vi "Main.vi"(11 "Module Admin":refnum<class "Delacor_lib_QMH_Module Admin.lvclass">) -> ()   [LabVIEW 2019, in "PF_trial_1.lvlib"]
doc: "This template is based off of the Queued Message Handler design pattern and the Queued Message Handler project template that ships with LabVIEW.\n\nThe main difference is that the queue is private to this module and communication between modules is performed via Broadcast and Request events.\n\nRequest events are wrapped in public API methods and are handled in the Event Handling Loop (EHL) of this VI. Any module can register for Broadcast events sent by this module. The EHL generates messages based on user interface actions.\n\nThe Message Handling Loop (MHL) processes messages generated by the EHL, or by other messages. The messages are string values, so new messages can be added easily to the Message Cases case structure in the MHL. Each message cluster can also provide an optional value for Message Data, which is a variant that can be converted to whatever message-specific data is required.\n_____\nBased on Delacor QMH Project Template 5.0.0.82."
uses:
  PF_trial_1.lvlib
  <vilib>/Delacor/Delacor QMH/Libraries/Module Admin_class/Delacor_lib_QMH_Module Admin.lvclass
  Module Data--cluster.ctl
  <vilib>/Delacor/Delacor QMH/Libraries/Message Queue_class/Delacor_lib_QMH_Message Queue.lvclass/Delacor_lib_QMH_Message Queue.ctl
  Stop Argument--cluster.ctl
  <vilib>/Delacor/Delacor QMH/Libraries/Module Admin_class/Delacor_lib_QMH_Module Admin.lvclass/Delacor_lib_QMH_Module Admin.ctl
  <vilib>/Utility/miscctls.llb/LVPointTypeDef.ctl
  <vilib>/Delacor/Delacor QMH/Libraries/Message Queue_class/Delacor_lib_QMH_Enqueue Message (Single).vi
  <vilib>/Delacor/Delacor QMH/Libraries/Module Admin_class/Delacor_lib_QMH_Get External Launch.vi
  <vilib>/Utility/error.llb/Error Cluster From Error Code.vi
  Global 1.vi
  <vilib>/ErrorRing/Error Ring.xnode
  <vilib>/Delacor/Delacor QMH/Libraries/Message Queue_class/Delacor_lib_QMH_Message Queue.lvclass
panel:
  out "Waveform Chart":dbl(graph)
  out "Gauge On?":bool
  in  "Get Status":bool
  in  "tpg361_delay":u32=50
  out "Error Status":string
  in  "Error status":bool
  out "Reset Status":string
  in  "Reset":bool
  in  "Gauge On-Off":enum16{"NO CHANGE", "OFF", "ON"}(ring)
  out "UNIT":string
  in  "Serial Settings:End Mode for Reads":u16(ring) items=["None", "Last Bit", "TermChar"]
  in  "Serial Settings:End Mode for Writes":u16(ring) items=["None", "Last Bit", "TermChar", "Break"]
  in  "Serial Settings:Baud Rate":u32(ring)=9600 items=["9.6KHz"=9600, "19.2KHz"=19200]
  in  "tpg_visa":refnum<visa-resource-name>
  out "Gauge Type":string
  in  "Get Gauge":bool
  in  "SETTING UNIT":T1(ring)=enum."Torr"
  in  "Acquisition time":i32=2000
  out "Pressure (Torr)":string
  in  "Get Pressure":bool
  in  "Simulate MHL Error":bool
  in  "Simulate EHL Error":bool
  out "error out":errorcluster
  out "Status":string
  # "RESET STATUS:\n0 = No Error\n1 = Watchdog has responded\n2 = Task Fail Error\n5 = FLASH Error\n6 = RAM Error\n7 = EEPROM Error\n9 = DISPLAY Error\n10 = A/D Converter Error\n11 = Gauge Error\n12 = Gauge Identification Error"
  # "ERROR STATUS:\n0000 = No Error\n1000 = ERROR (controller error (see display on front\npanel)\n0100 = NO HWR (no hardware) \n0010 = PAR (inadmissible parameter) \n0001 = SYN (Syntax error)"
  # "INITIALIZATION:"
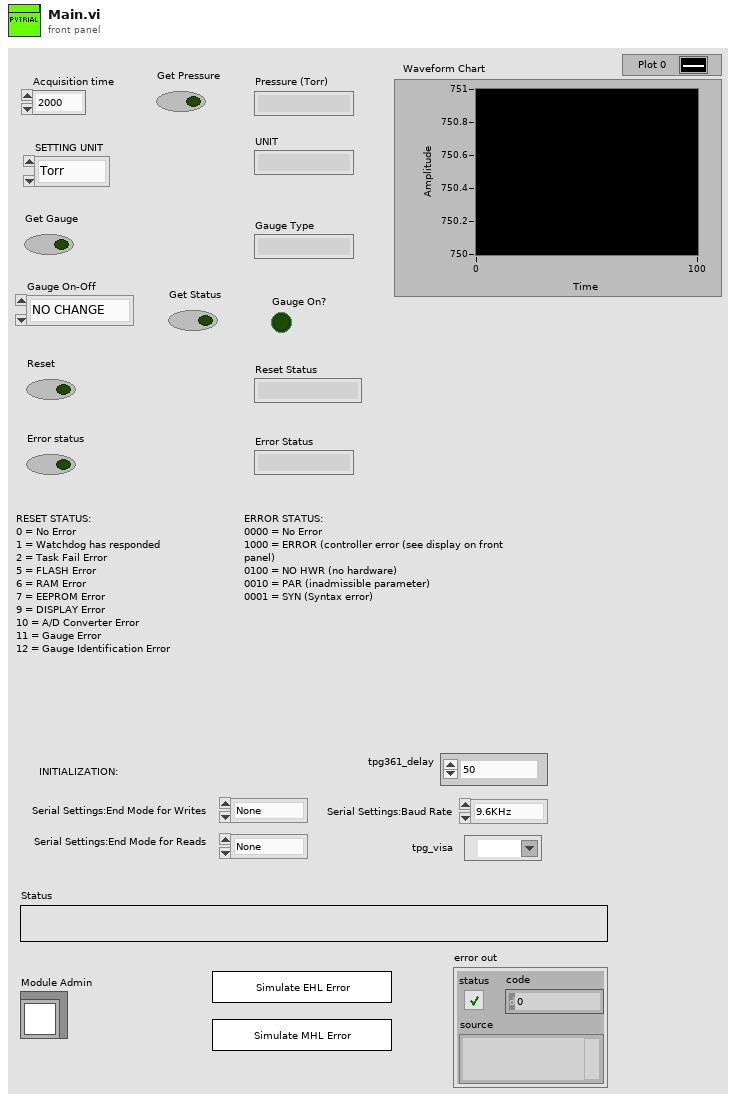
[diagram p1: front panel]
types:
  T1 = enum16{"mBar", "Torr", "Pascal", "micron", "hPascal", "Volt"}
  T2 = typedef "PF_trial_1.lvlib/Request Events--cluster.ctl" = cluster{"Stop Module":refnum<user-event>, "Show Panel":refnum<user-event>, "Hide Panel":refnum<user-event>, "Get Module Execution Status":refnum<user-event>, "Show Diagram":refnum<user-event>}
  T3 = typedef "PF_trial_1.lvlib/Module Data--cluster.ctl" = cluster{"Status":string}
  T4 = enum32{"invalid lock state", "Not Locked", "Locked (No Password)", "Password-protected"}
  T5 = typedef "PF_trial_1.lvlib/Stop Argument--cluster.ctl" = cluster{"Origin":string, "Exit via Stop Module Req?":bool, "Wait for Module to stop?":bool}
  T6 = typedef "LVPointTypeDef.ctl" = cluster{"Horizontal":i16, "Vertical":i16}
  T7 = enum32{"Invalid", "Standard", "Closed", "Hidden", "Minimized", "Maximized"}
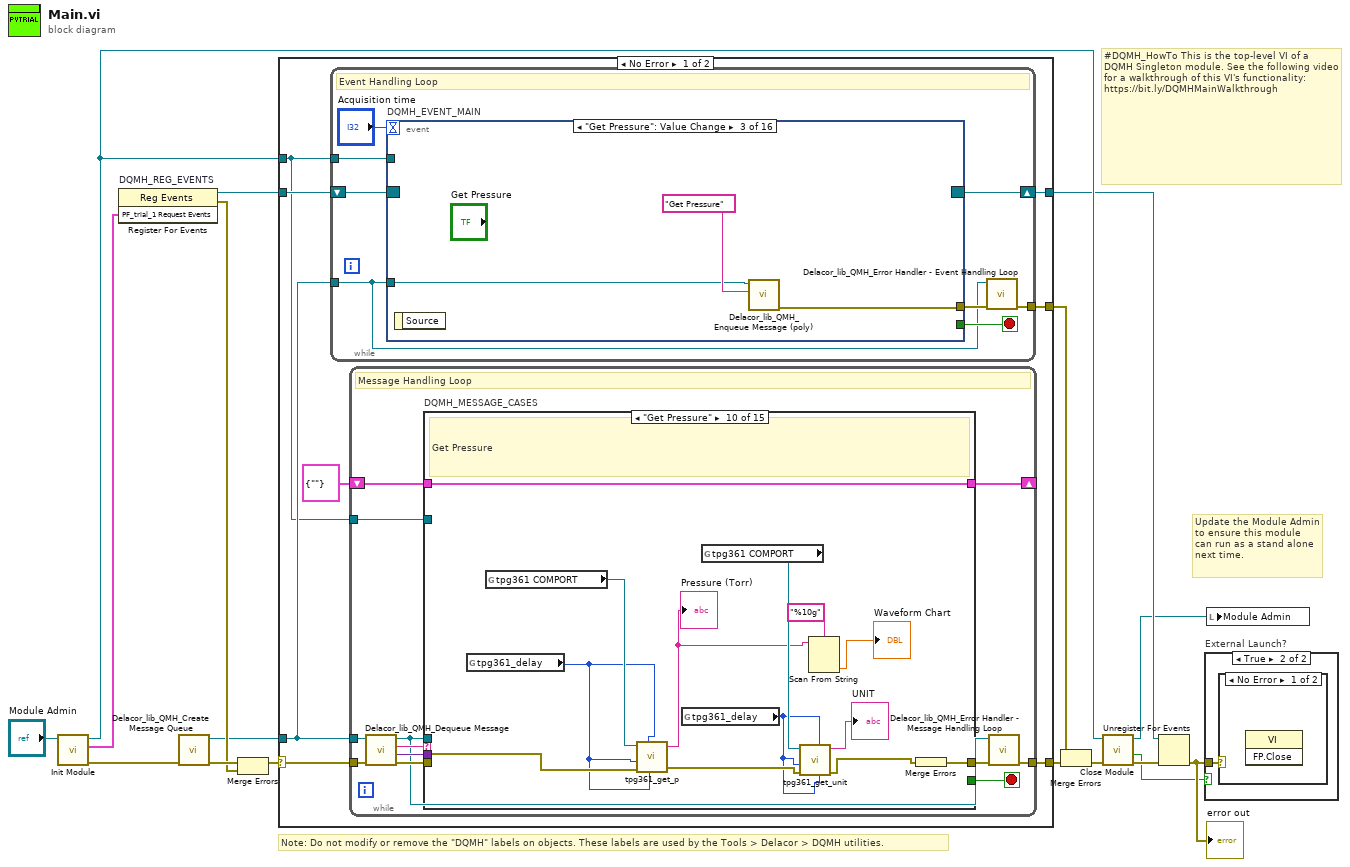
[diagram p0: block diagram]
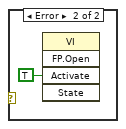
[diagram p3: hidden frame]
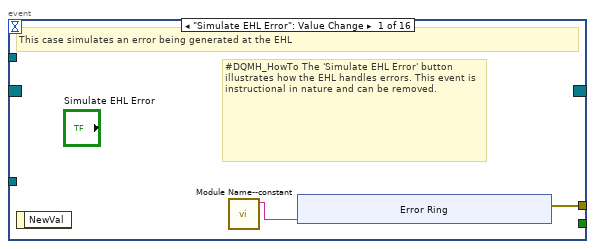
[diagram p4: hidden frame]
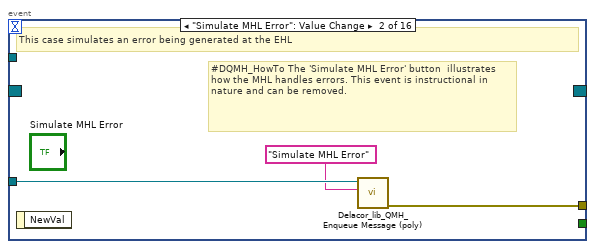
[diagram p5: hidden frame]
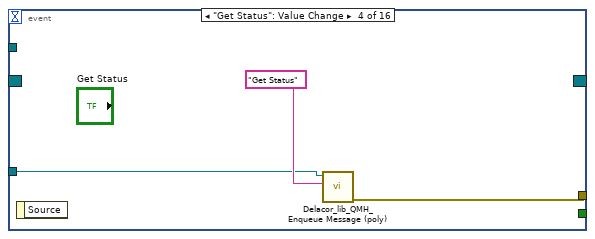
[diagram p6: hidden frame]
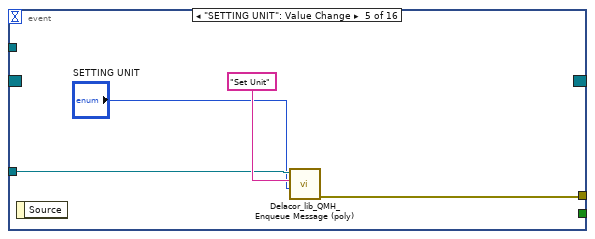
[diagram p7: hidden frame]
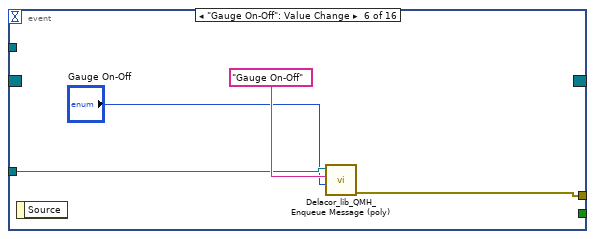
[diagram p8: hidden frame]
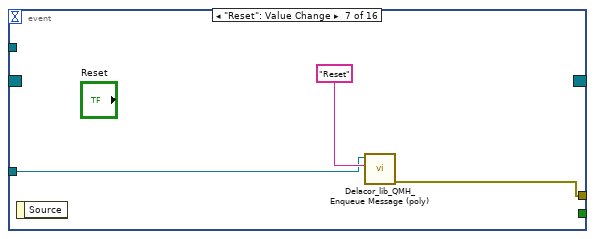
[diagram p9: hidden frame]
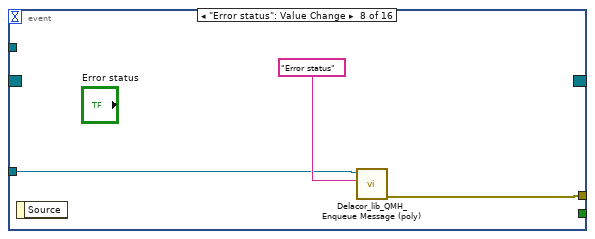
[diagram p10: hidden frame]
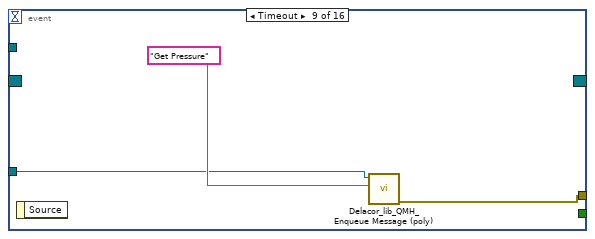
[diagram p11: hidden frame]
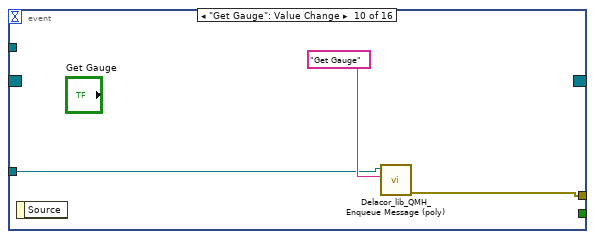
[diagram p12: hidden frame]
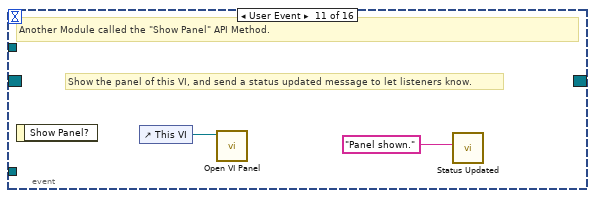
[diagram p13: hidden frame]
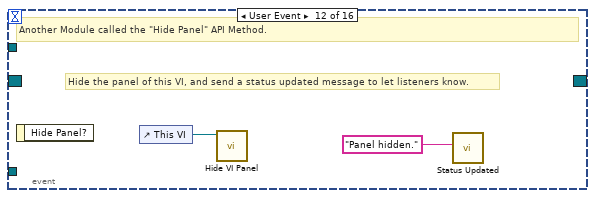
[diagram p14: hidden frame]
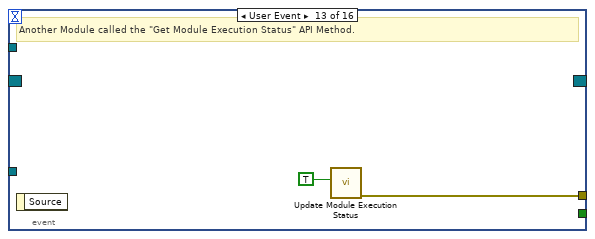
[diagram p15: hidden frame]
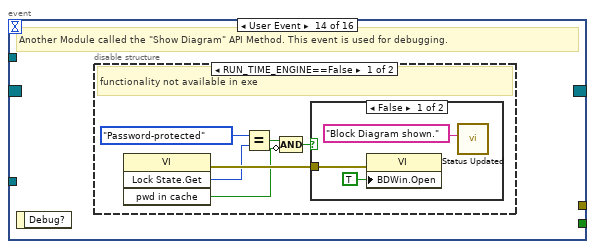
[diagram p16: hidden frame]
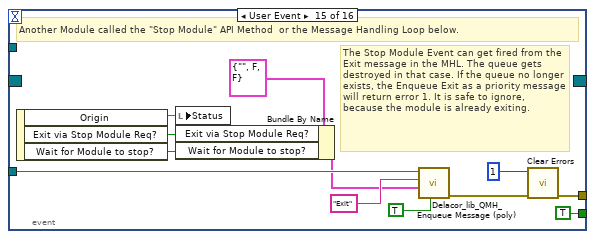
[diagram p19: hidden frame]
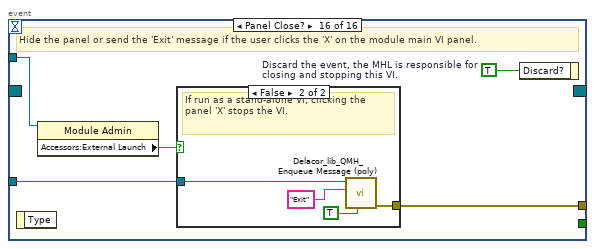
[diagram p20: hidden frame]
diagram:
  # "#DQMH_HowTo This is the top-level VI of a DQMH Singleton module. See the following video for a walkthrough of this VI's functionality: https://bit.ly/DQMHMainWalkthrough"
  # "Note: Do not modify or remove the \"DQMH\" labels on objects. These labels are used by the Tools > Delacor > DQMH utilities."
  # "Update the Module Admin to ensure this module can run as a stand alone next time."
  n1 = call "Init Module.vi"("Singleton Module Admin in"="Module Admin") -> ("error out"=w16:errorcluster, "PF_trial_1 Request Events"=w5:T2, "Singleton Module Admin out"=w8:refnum<class "Delacor_lib_QMH_Module Admin.lvclass">)  [unwired: 8 in]
  n2 = register-events "DQMH_REG_EVENTS"(w5) -> (reference out=w6:refnum<event-registration>, error out=w9:errorcluster)  [unwired: 2 in]
  n3 = call <vilib>:"Delacor_lib_QMH_Create Message Queue.vi"("error in (no error)"=w16) -> ("error out"=w11:errorcluster, "Message Queue"=w4:refnum<class "Delacor_lib_QMH_Message Queue.lvclass">)  [unwired: 9 in]
  n4 = Merge Errors(w11, w9) -> (w10:errorcluster)
  n5 = case shown="No Error" w10 {
    selector: w10 -> [w23 w273]
    tunnel: [w25 w272] -> w17
    tunnel: [w22 w278] -> w7
    tunnel: w6 -> [w20 w278]
    tunnel: w4 -> [w19 w271]
    tunnel: [w24 _] -> w14
    tunnel: w8 -> [w18 w274]
    frame No Error {
      n6 = while {
        tunnel: w19 -> [w27]
        shift-right: [w30] -> w22
        shift-left: w20 -> [w31]
        tunnel: [w32] -> w24
        tunnel: w18 -> [w28]
        stop <- w29 stop-if-true
        # "Event Handling Loop"
        n7 = event "DQMH_EVENT_MAIN" shown="[2] \"Get Pressure\": Value Change" {
          selector: w31 -> [_ _ _ _ _ _ _ _ _ _ _ _ _ _ _ _]
          dyn-events: [_ _ _ _ _ _ _ _ _ _ _ _ _ _ _ _] -> w30
          timeout: "Acquisition time" -> [_ _ _ _ _ _ _ _ _ _ _ _ _ _ _ _]
          tunnel: [_ _ _ _ _ _ _ _ _ _ _ _ _ _ TRUE ("Discard?") _] -> w29
          tunnel: w27 -> [_ w44 w47 w50 w54 w58 w60 w64 w67 w70 _ _ _ _ w94 w101]
          tunnel: [w35 w45 w46 w49 w53 w56 w61 w63 w66 w69 _ _ w77 _ w97 w103] -> w33
          tunnel: w28 -> [_ _ _ _ _ _ _ _ _ _ _ _ _ _ _ w100]
          event "Simulate EHL Error": Value Change {
            # "#DQMH_HowTo The 'Simulate EHL Error' button  illustrates how the EHL handles errors. This event is instructional in nature and can be removed."
            # "This case simulates an error being generated at the EHL"
            n8 = event-data() -> ()  [unwired: 1 in, 1 out]
            n9 = call "Module Name--constant.vi"() -> ("Module Name"=w34:string)  [unwired: 11 in]
            n10 = xnode "Error Ring"("parameter 0"=w34) -> ("error out"=w35:errorcluster)
          }
          event "Simulate MHL Error": Value Change {
            # "#DQMH_HowTo The 'Simulate MHL Error' button  illustrates how the MHL handles errors. This event is instructional in nature and can be removed."
            # "This case simulates an error being generated at the EHL"
            n11 = event-data() -> ()  [unwired: 1 in, 1 out]
            n12 = call-poly <vilib>:"Delacor_lib_QMH_Enqueue Message (poly).vi"("Message"="Simulate MHL Error", "Message Queue in"=w44) -> ("error out"=w45:errorcluster)  [unwired: 8 in, 1 out]
          }
          event "Get Pressure": Value Change {
            n13 = event-data() -> ()  [unwired: 1 in, 1 out]
            n14 = call-poly <vilib>:"Delacor_lib_QMH_Enqueue Message (poly).vi"("Message"="Get Pressure", "Message Queue in"=w47) -> ("error out"=w46:errorcluster)  [unwired: 8 in, 1 out]
          }
          event "Get Status": Value Change {
            n15 = event-data() -> ()  [unwired: 1 in, 1 out]
            n16 = call-poly <vilib>:"Delacor_lib_QMH_Enqueue Message (poly).vi"("Message"="Get Status", "Message Queue in"=w50) -> ("error out"=w49:errorcluster)  [unwired: 8 in, 1 out]
          }
          event "SETTING UNIT": Value Change {
            n17 = event-data() -> ()  [unwired: 1 in, 1 out]
            n18 = call-poly <vilib>:"Delacor_lib_QMH_Enqueue Message (poly).vi"("Message Data"="SETTING UNIT", "Message"="Set Unit", "Message Queue in"=w54) -> ("error out"=w53:errorcluster)  [unwired: 7 in, 1 out]
          }
          event "Gauge On-Off": Value Change {
            n19 = event-data() -> ()  [unwired: 1 in, 1 out]
            n20 = call-poly <vilib>:"Delacor_lib_QMH_Enqueue Message (poly).vi"("Message Data"="Gauge On-Off", "Message"="Gauge On-Off", "Message Queue in"=w58) -> ("error out"=w56:errorcluster)  [unwired: 7 in, 1 out]
          }
          event "Reset": Value Change {
            n21 = event-data() -> ()  [unwired: 1 in, 1 out]
            n22 = call-poly <vilib>:"Delacor_lib_QMH_Enqueue Message (poly).vi"("Message"="Reset", "Message Queue in"=w60) -> ("error out"=w61:errorcluster)  [unwired: 8 in, 1 out]
          }
          event "Error status": Value Change {
            n23 = event-data() -> ()  [unwired: 1 in, 1 out]
            n24 = call-poly <vilib>:"Delacor_lib_QMH_Enqueue Message (poly).vi"("Message"="Error status", "Message Queue in"=w64) -> ("error out"=w63:errorcluster)  [unwired: 8 in, 1 out]
          }
          event Timeout {
            n25 = event-data() -> ()  [unwired: 1 in, 1 out]
            n26 = call-poly <vilib>:"Delacor_lib_QMH_Enqueue Message (poly).vi"("Message"="Get Pressure", "Message Queue in"=w67) -> ("error out"=w66:errorcluster)  [unwired: 8 in, 1 out]
          }
          event "Get Gauge": Value Change {
            n27 = event-data() -> ()  [unwired: 1 in, 1 out]
            n28 = call-poly <vilib>:"Delacor_lib_QMH_Enqueue Message (poly).vi"("Message"="Get Gauge", "Message Queue in"=w70) -> ("error out"=w69:errorcluster)  [unwired: 8 in, 1 out]
          }
          event User Event {
            # "Show the panel of this VI, and send a status updated message to let listeners know."
            # "Another Module called the \"Show Panel\" API Method."
            n29 = event-data() -> ()  [unwired: 1 in, 1 out]
            n30 = control-ref of="This VI"() -> (w73:refnum<vi>)
            n31 = call "Open VI Panel.vi"("VI"=w73) -> ()  [unwired: 10 in, 1 out]
            n32 = call "Status Updated.vi"("Status"="Panel shown." ("format string")) -> ()  [unwired: 10 in, 1 out]
          }
          event User Event {
            # "Hide the panel of this VI, and send a status updated message to let listeners know."
            # "Another Module called the \"Hide Panel\" API Method."
            n33 = event-data() -> ()  [unwired: 1 in, 1 out]
            n34 = control-ref of="This VI"() -> (w75:refnum<vi>)
            n35 = call "Hide VI Panel.vi"("VI"=w75) -> ()  [unwired: 10 in, 1 out]
            n36 = call "Status Updated.vi"("Status"="Panel hidden." ("format string")) -> ()  [unwired: 10 in, 1 out]
          }
          event User Event {
            # "Another Module called the \"Get Module Execution Status\" API Method."
            n37 = event-data() -> ()  [unwired: 1 in, 1 out]
            n38 = call "Update Module Execution Status.vi"("Running?"=TRUE) -> ("error out"=w77:errorcluster)  [unwired: 10 in]
          }
          event User Event {
            # "Another Module called the \"Show Diagram\" API Method. This event is used for debugging."
            n39 = event-data() -> ()  [unwired: 1 in, 1 out]
            n40 = disable-structure shown="RUN_TIME_ENGINE==False" {
              frame condition #0 (active) {
                # "functionality not available in exe"
                n41 = invoke class="VI" method="Lock State.Get"() -> (error out=w83:errorcluster, "Get Lock State"=w82:T4, "pwd in cache"=w79:bool)  [unwired: 4 in, 1 out]
                n42 = Equal?(x=T4."Password-protected", y=w82) -> (x = y?=w80:bool)
                n43 = Compound Arithmetic op=AND(w80, invert w79) -> (w78:bool)
                n44 = case shown="False" w78 {
                  tunnel: w83 -> [w86 _]
                  frame False {
                    n45 = property class="VI"(error in=w86, "BDWin.Open"=TRUE ("Block Diagram Window:Open")) -> ()  [unwired: 1 in, 2 out]
                    n46 = call "Status Updated.vi"("Status"="Block Diagram shown." ("format string")) -> ()  [unwired: 10 in, 1 out]
                  }
                  frame True {
                    # "Password-protected VI, and the password is not in the cache. Do not show the diagram."
                  }
                }
              }
              frame condition #1 {
              }
            }
          }
          event User Event {
            # "The Stop Module Event can get fired from the Exit message in the MHL. The queue gets destroyed in that case. If the queue no longer exists, the Enqueue Exit as a priority message will return error 1. It is safe to ignore, because the module is already exiting."
            # "Another Module called the \"Stop Module\" API Method  or the Message Handling Loop below."
            n47 = event-data() -> ("Origin"=w93:string, "Exit via Stop Module Req?"=w89:bool, "Wait for Module to stop?"=w88:bool)  [unwired: 1 in]
            n48 = local write "Status"(w93) -> ()
            n49 = Bundle By Name(cluster=T5 {"Origin"="", "Exit via Stop Module Req?"=FALSE, "Wait for Module to stop?"=FALSE} ("Stop Argument"), "Exit via Stop Module Req?"=w89, "Wait for Module to stop?"=w88) -> (w87:T5)
            n50 = call-poly <vilib>:"Delacor_lib_QMH_Enqueue Message (poly).vi"("Priority Message? (F)"=TRUE, "Message Data"=w87, "Message"="Exit", "Message Queue in"=w94) -> ("error out"=w98:errorcluster)  [unwired: 6 in, 1 out]
            n51 = call <vilib>:"Clear Errors.vi"("error in (no error)"=w98, "specific error code to clear (0: all)"=1) -> ("error out"=w97:errorcluster)  [unwired: 4 in, 1 out]
          }
          event Panel Close? {
            w102 = TRUE  # Discard the event, the MHL is responsible for closing and stopping this VI.
            # "Hide the panel or send the 'Exit' message if the user clicks the 'X' on the module main VI panel."
            n52 = event-data() -> ()  [unwired: 1 in, 1 out]
            n53 = property class="Module Admin"(reference=w100) -> ("Accessors:External Launch"=w99:bool)  [unwired: 1 in, 2 out]
            n54 = case shown="False" w99 {
              tunnel: w101 -> [_ w107]
              tunnel: [_ w108] -> w103
              frame True {
                # "If externally launched, clicking the 'X' hides the panel, but doesn't close it."
                n55 = control-ref of="This VI"() -> (w104:refnum<vi>)
                n56 = call "Hide VI Panel.vi"("VI"=w104) -> ()  [unwired: 10 in, 1 out]
              }
              frame False {
                # "If run as a stand-alone VI, clicking the panel 'X' stops the VI."
                n57 = call-poly <vilib>:"Delacor_lib_QMH_Enqueue Message (poly).vi"("Priority Message? (F)"=TRUE, "Message"="Exit", "Message Queue in"=w107) -> ("error out"=w108:errorcluster)  [unwired: 7 in, 1 out]
              }
            }
            n58 = event-data("Discard?"=w102) -> ()  [unwired: 1 in, 1 out]
          }
        }
        n59 = call-dynamic "Delacor_lib_QMH_Error Handler - Event Handling Loop.vi"("error in (no error)"=w33, "Message Queue in"=w27) -> ("dup error in"=w32:errorcluster)  [unwired: 8 in, 1 out]
      }
      n60 = while {
        tunnel: w19 -> [w111]
        shift-right: [w115] -> _
        shift-left: T3 {"Status"=""} ("Data Cluster") -> [w116]
        tunnel: w23 -> [w119]
        tunnel: [w117] -> w25
        tunnel: w18 -> [w109]
        stop <- w114 stop-if-true
        # "Message Handling Loop"
        n61 = call-dynamic "Delacor_lib_QMH_Dequeue Message.vi"("error in (no error)"=w119, "Message Queue in"=w111) -> ("error out"=w118:errorcluster, "Message Data"=w112:variant, "Message"=w113:string, "Message Queue out"=w110:refnum<class "Delacor_lib_QMH_Message Queue.lvclass">)  [unwired: 6 in]
        n62 = case "DQMH_MESSAGE_CASES" shown="\"Get Pressure\"" w113 {
          selector: w113 -> [_ _ _ _ _ _ _ _ _ _ _ _ _ _ w258]
          tunnel: w110 -> [_ _ _ _ _ _ _ _ _ _ _ _ w226 w251 _]
          tunnel: w118 -> [w144 w148 w151 w154 w162 w168 w177 w183 w192 w206 w210 w215 w233 w256 w260]
          tunnel: [w143 w148 w150 w158 w164 w170 w179 w185 w195 w208 w210 w214 w229 w254 w261] -> w120
          tunnel: w116 -> [w134 w147 w149 w157 w163 w169 w178 w184 w194 w207 w209 w212 w228 w250 w259]
          tunnel: [w133 w147 w149 w157 w163 w169 w178 w184 w194 w207 w209 w212 w228 w250 w259] -> w115
          tunnel: [_ _ _ _ _ _ _ _ _ _ _ _ _ w249 _] -> w114
          tunnel: w112 -> [_ _ _ _ _ _ w174 _ w190 _ _ _ w227 w248 _]
          tunnel: w109 -> [w135 _ _ _ _ _ _ _ _ _ _ _ w225 w243 _]
          frame "Initialize" {
            w128 = "Initial Message" ("Initial Message")
            # "#CodeNeeded - Initialize the appearance of the front panel."
            # "Initialize - Any operation that needs to be done before the module can receive messages. Synchronize Caller Events.vi will inform Start Module.vi that the module has launched and is ready to receive messages. Module Did Init.vi will broadcast that the module initialized."
            n63 = call "Synchronize Caller Events.vi"("error in (no error)"=w144, "Singleton Module Admin in"=w135) -> ("error out"=w127:errorcluster, "Singleton Module Admin out"=w130:refnum<class "Delacor_lib_QMH_Module Admin.lvclass">)  [unwired: 8 in]
            n64 = property class="Module Admin"(reference=w130) -> ("Accessors:External Launch"=w139:bool)  [unwired: 1 in, 2 out]
            n65 = global write "Global 1.vi" "tpg361_delay"("tpg361_delay") -> ()
            n66 = global write "Global 1.vi" "tpg361 COMPORT"("tpg_visa") -> ()
            n67 = Select(t=T7."Hidden" ("State"), s=w139, f=T7."Standard" ("State")) -> (s? t:f=w136:T7)
            n68 = call "tpg361_visa_init.vi"("thcd_visa"="tpg_visa", "err_in"=w127, "Serial Settings:Baud Rate"="Serial Settings:Baud Rate", "Serial Settings:End Mode for Writes"="Serial Settings:End Mode for Writes", "Serial Settings:End Mode for Reads"="Serial Settings:End Mode for Reads") -> ("err_out"=w126:errorcluster)  [unwired: 1 out]
            n69 = call "Module Name--constant.vi"() -> ("Module Name"=w142:string)  [unwired: 11 in]
            n70 = property class="VI"("Front Panel.Title"=w142) -> (reference out=w141:refnum<vi>, error out=w146:errorcluster)  [unwired: 2 in]
            n71 = call "Module Name--constant.vi"() -> ("Module Name"=w131:string)  [unwired: 11 in]
            n72 = invoke class="VI" method="FP.Open"(reference=w141, error in=w146, "State"=w136) -> (reference out=w140:refnum<vi>, error out=w145:errorcluster)  [unwired: 2 in, 3 out]
            n73 = Bundle By Name(cluster=w134, "Status"=w128) -> (w133:T3)
            n74 = call "Module Did Init.vi"("error in (no error)"=w126, "Initialized?"=TRUE, "Origin"=w131) -> ("error out"=w143:errorcluster)  [unwired: 8 in]
            n75 = invoke class="VI" method="FP.Center"(reference=w140, error in=w145) -> ()  [unwired: 1 in, 3 out]
            n76 = property on="Pane" class="Pane"("Origin"=T6 {"Horizontal"=0, "Vertical"=0}) -> ()  [unwired: 2 in, 2 out]
            "Status" <- w128
          }
          frame "--- Module Specific ---" {
            # "Separator -- The following cases handle messages specific to this Module."
          }
          frame "---Copy This Frame---" {
            # "Duplicate this frame when creating new messages.  Change this comment in the duplicated frame to describe this message."
            n77 = Merge Errors(w151) -> (w150:errorcluster)
          }
          frame "Get Status" {
            # "Duplicate this frame when creating new messages.  Change this comment in the duplicated frame to describe this message."
            n78 = global read "Global 1.vi" "tpg361 COMPORT"() -> (w155:refnum<visa-resource-name>)
            n79 = global read "Global 1.vi" "tpg361_delay"() -> (w152:u32)
            n80 = call "tpg361_get_status.vi"("tpg361_delay 3"=w152, "tpg361_delay 2"=w152, "err_in"=w154, "tpg361_delay"=w152, "tpg361_visa"=w155) -> ("err_out"=w153:errorcluster, "Gauge status"=→"Gauge On?":bool)  [unwired: 4 in]
            n81 = Merge Errors(w153) -> (w158:errorcluster)
          }
          frame "Error status" {
            # "Duplicate this frame when creating new messages.  Change this comment in the duplicated frame to describe this message."
            n82 = global read "Global 1.vi" "tpg361 COMPORT"() -> (w160:refnum<visa-resource-name>)
            n83 = call "tpg361_ERR.vi"("err_in"=w162, "tpg361_visa"=w160) -> ("err_out"=w161:errorcluster, "Error Status"=→"Error Status":string)  [unwired: 7 in]
            n84 = Merge Errors(w161) -> (w164:errorcluster)
          }
          frame "Reset" {
            # "Duplicate this frame when creating new messages.  Change this comment in the duplicated frame to describe this message."
            n85 = global read "Global 1.vi" "tpg361 COMPORT"() -> (w166:refnum<visa-resource-name>)
            n86 = call "tpg361_reset.vi"("err_in"=w168, "tpg361_visa"=w166) -> ("err_out"=w167:errorcluster, "Error Status"=→"Reset Status":string)  [unwired: 7 in]
            n87 = Merge Errors(w167) -> (w170:errorcluster)
          }
          frame "Gauge On-Off" {
            # "Duplicate this frame when creating new messages.  Change this comment in the duplicated frame to describe this message."
            n88 = Variant To Data(error in=w177, Variant=w174) -> (data=w173:enum16{"NO CHANGE", "OFF", "ON"}, error out=w176:errorcluster)  [unwired: 1 in]
            n89 = global read "Global 1.vi" "tpg361_delay"() -> (w172:u32)
            n90 = global read "Global 1.vi" "tpg361 COMPORT"() -> (w175:refnum<visa-resource-name>)
            n91 = call "tpg361_on_off.vi"("tpg361_delay 3"=w172, "tpg361_delay 2"=w172, "err_in"=w176, "tpg361_delay"=w172, "Gauge On-Off"=w173, "tpg361_visa"=w175) -> ("err_out"=w171:errorcluster)  [unwired: 3 in, 1 out]
            n92 = Merge Errors(w171) -> (w179:errorcluster)
          }
          frame "Get Gauge" {
            # "Duplicate this frame when creating new messages.  Change this comment in the duplicated frame to describe this message."
            n93 = global read "Global 1.vi" "tpg361 COMPORT"() -> (w180:refnum<visa-resource-name>)
            n94 = call "tpg361_get_gauge.vi"("err_in"=w183, "tpg361_visa"=w180) -> ("err_out"=w182:errorcluster, "Gauge Type"=→"Gauge Type":string)  [unwired: 7 in]
            n95 = Merge Errors(w182) -> (w185:errorcluster)
          }
          frame "Set Unit" {
            # "Set Unit"
            n96 = global read "Global 1.vi" "tpg361_delay"() -> (w186:u32)
            n97 = Variant To Data(error in=w192, type=T1."Torr", Variant=w190) -> (data=w189:T1, error out=w191:errorcluster)
            n98 = global read "Global 1.vi" "tpg361 COMPORT"() -> (w187:refnum<visa-resource-name>)
            n99 = call "tpg361_set_unit.vi"("tpg361_delay 3"=w186, "tpg361_delay 2"=w186, "err_in"=w191, "tpg361_delay"=w186, "tpg361_visa"=w187, "SETTING UNIT"=w189) -> ("err_out"=w193:errorcluster)  [unwired: 4 in]
            n100 = Merge Errors(w193) -> (w195:errorcluster)
          }
          frame "Get Pressure" {
            # "Get Pressure"
            n101 = global read "Global 1.vi" "tpg361_delay"() -> (w204:u32)
            n102 = global read "Global 1.vi" "tpg361 COMPORT"() -> (w205:refnum<visa-resource-name>)
            n103 = call "tpg361_get_p.vi"("tpg361_delay 3"=w204, "err_in"=w206, "tpg361_delay"=w204, "tpg361_delay 2"=w204, "tpg361_visa"=w205) -> ("err_out"=w203:errorcluster, "Pressure (Torr)"=w198:string)  [unwired: 4 in]
            "Pressure (Torr)" <- w198
            n104 = global read "Global 1.vi" "tpg361_delay"() -> (w200:u32)
            n105 = global read "Global 1.vi" "tpg361 COMPORT"() -> (w201:refnum<visa-resource-name>)
            n106 = call "tpg361_get_unit.vi"("tpg361_visa"=w201, "tpg361_delay"=w200, "err_in"=w203, "tpg361_delay 2"=w200, "tpg361_delay 3"=w200) -> ("UNIT"=→"UNIT":string, "err_out"=w202:errorcluster)  [unwired: 3 in]
            n107 = Scan From String(format string="%10g", input string=w198) -> (output 1=→"Waveform Chart":dbl)  [unwired: 3 in, 3 out]
            n108 = Merge Errors(w202) -> (w208:errorcluster)
          }
          frame "--- Exit and Error Handling---" {
            # "Separator - The following cases handle errors and exit messages."
          }
          frame "Simulate MHL Error" {
            # "#DQMH_HowTo The 'Simulate MHL Error' button  illustrates how the MHL handles errors. This event is instructional in nature and can be removed."
            # "Simulate an error occurring at the MHL"
            n109 = call "Module Name--constant.vi"() -> ("Module Name"=w211:string)  [unwired: 11 in]
            n110 = xnode "Error Ring"("parameter 0"=w211) -> ("error out"=w213:errorcluster)
            n111 = Merge Errors(w215, w213) -> (w214:errorcluster)
          }
          frame "Error" {
            # "#CodeRecommended - If you ever change the name of this \"Error\" message, you'll need to update the name in the Check Loop Error.vi as well."
            # "#CodeRecommended - If the module is running in standalone mode (External Launch = FALSE), this code will pop up an error dialog and call the 'Exit' message if an error occurs. Add more fine-grained error handling here."
            # "Error - Check the error message data and respond accordingly. This message is sent by the \"Error Handler\" VIs at the end of each loop in this application."
            n112 = property class="Module Admin"(reference=w225) -> ("Accessors:External Launch"=w224:bool)  [unwired: 1 in, 2 out]
            n113 = Variant To Data(error in=w233, type=errorcluster {"status"=FALSE, "code"=0, "source"=""} ("error constant"), Variant=w227) -> (data=w234:errorcluster, error out=w231:errorcluster)
            n114 = call "Module Name--constant.vi"() -> ("Module Name"=w223:string)  [unwired: 11 in]
            n115 = call "Error Reported.vi"("Additional Information"=w223, "Error"=w234) -> ()  [unwired: 9 in, 1 out]
            n116 = case shown="False" w224 {
              tunnel: [w239 _] -> w230
              tunnel: w226 -> [w237 _]
              tunnel: w234 -> [w238 _]
              frame False {
                # "If the module is running standalone, then pop up an error dialog and call the \"Exit\" message."
                n117 = call <vilib>:"Simple Error Handler.vi"("error in (no error)"=w238) -> ()  [unwired: 4 in, 5 out]
                n118 = call-poly <vilib>:"Delacor_lib_QMH_Enqueue Message (poly).vi"("Priority Message? (F)"=TRUE, "Message"="Exit", "Message Queue in"=w237) -> ("error out"=w239:errorcluster)  [unwired: 7 in, 1 out]
              }
              frame True {
                # "If the module was launched externally, calling the Error Reported broadcast VI is the only action performed by the \"Error\" message. The module's caller can then process the error appropriately."
              }
            }
            n119 = Merge Errors(w231, w230) -> (w229:errorcluster)
            n120 = local write "error out"(w229) -> ()
          }
          frame "Exit" {
            w247 = 91  # 91: not all Exit messages will have an argument
            w249 = TRUE  # Stop the VI
            # "Release the message queue reference"
            # "#CodeNeeded - Add any required cleanup code here"
            # "Exit - Exit the application."
            n121 = Variant To Data(error in=w256, type=T5 {"Origin"="", "Exit via Stop Module Req?"=FALSE, "Wait for Module to stop?"=FALSE} ("Stop Argument"), Variant=w248) -> (data=w245:T5, error out=w253:errorcluster)
            n122 = call <vilib>:"Clear Errors.vi"("error in (no error)"=w253, "specific error code to clear (0: all)"=w247) -> ("error out"=w255:errorcluster)  [unwired: 4 in, 1 out]
            n123 = global read "Global 1.vi" "tpg361 COMPORT"() -> (w240:refnum<visa-resource-name>)
            n124 = call-dynamic "Delacor_lib_QMH_Release Message Queue.vi"("error in (no error)"=w255, "Message Queue"=w251) -> ("error out"=w242:errorcluster)  [unwired: 9 in]
            n125 = control-ref of="This VI"() -> (w244:refnum<vi>)
            n126 = call "tpg361_visa_close.vi"("VISA session"=w240, "error in (no error)"=w242) -> ("error out"=w241:errorcluster)  [unwired: 13 in]
            n127 = call "Handle Exit.vi"("Stop Argument"=w245, "Admin in"=w243, "VI reference"=w244) -> ("error out"=w252:errorcluster)  [unwired: 7 in, 1 out]
            n128 = Merge Errors(w241, w252) -> (w254:errorcluster)
          }
          frame Default {
            # "'Default' case only runs if there is a message that isn't defined in any of the other cases.  Output a programming error."
            n129 = call "Module Name--constant.vi"() -> ("Module Name"=w257:string)  [unwired: 11 in]
            n130 = xnode "Error Ring"("parameter 0"=w258, "parameter 1"=w257) -> ("error out"=w262:errorcluster)
            n131 = Merge Errors(w260, w262) -> (w261:errorcluster)
          }
        }
        n132 = call-dynamic "Delacor_lib_QMH_Error Handler - Message Handling Loop.vi"("error in (no error)"=w120, "Message Queue in"=w110) -> ("dup error in"=w117:errorcluster)  [unwired: 8 in, 1 out]
      }
    }
    frame Error {
      # "Synchronize Caller Events.vi will inform Start Module.vi that the module has launched and will let the code calling Start Module.vi register for broadcasts and would permit the caller receive the broadcast that an error occurred at launch time."
      n133 = call-dynamic "Delacor_lib_QMH_Release Message Queue.vi"("error in (no error)"=w273, "Message Queue"=w271) -> ("error out"=w272:errorcluster)  [unwired: 9 in]
      n134 = call "Synchronize Caller Events.vi"("Singleton Module Admin in"=w274) -> ("error out"=w279:errorcluster)  [unwired: 9 in, 1 out]
      n135 = call "Module Name--constant.vi"() -> ("Module Name"=w277:string)  [unwired: 11 in]
      n136 = Format Into String(format string="An error occurred during initialization. %s is no longer running.", w277) -> (resulting string=w275:string)  [unwired: 2 in, 1 out]
      n137 = Merge Errors(w272, w279) -> (w280:errorcluster)
      n138 = call "Error Reported.vi"("Additional Information"=w275, "Error"=w280) -> ()  [unwired: 9 in, 1 out]
    }
  }
  n139 = Merge Errors(w14, w17) -> (w13:errorcluster)
  n140 = call "Close Module.vi"("error in (no error)"=w13, "Module Admin in"=w8) -> ("error out"=w15:errorcluster, "External Launch"=w1:bool, "Module Admin out"=w2:refnum<class "Delacor_lib_QMH_Module Admin.lvclass">)  [unwired: 7 in]
  n141 = Unregister For Events(event registration refnum=w7, error in=w15) -> (error out=w12:errorcluster)
  "error out" <- w12
  n142 = case "External Launch?" shown="True" w1 {
    tunnel: w12 -> [_ w281]
    frame False {
    }
    frame True {
      n143 = case shown="No Error" w281 {
        frame No Error {
          n144 = invoke class="VI" method="FP.Close"() -> ()  [unwired: 3 in, 3 out]
        }
        frame Error {
          n145 = invoke class="VI" method="FP.Open"("Activate"=TRUE ("Activate?")) -> ()  [unwired: 4 in, 5 out]
        }
      }
    }
  }
  n146 = local write "Module Admin"(w2) -> ()
